vi "SC FPGA.vi"() -> ()   [LabVIEW 2015]
uses:
  <vilib>/eio/EIONode/EIONode.xnode
  <vilib>/rvi/eio/common/nirviEmuTemplateMethod_errors.vi
panel:
  out "Encoder Position":i32
  out "Converted Encoder":bool[](array[boolean])
  out "Raw Encoder":bool[](array[boolean])
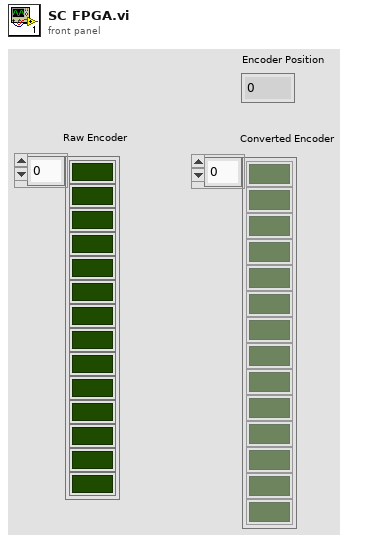
[diagram p1: front panel]
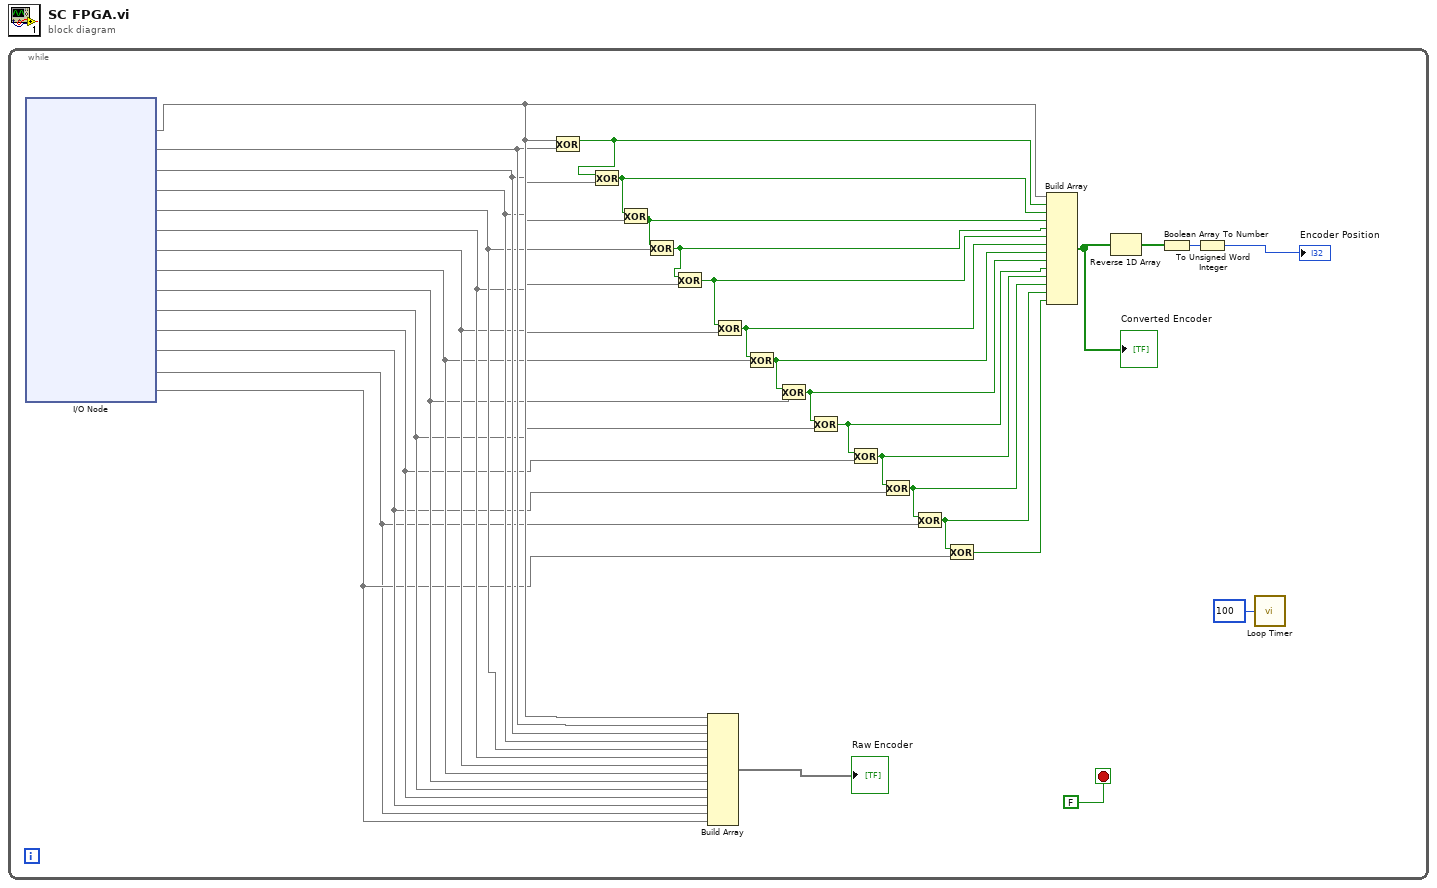
[diagram p0: block diagram]
diagram:
  n1 = while {
    stop <- FALSE stop-if-true
    n2 = xnode "I/O Node"() -> ("Mod6/DIO13"=w15, "Mod6/DIO12"=w14, "Mod6/DIO11"=w13, "Mod6/DIO10"=w12, "Mod6/DIO9"=w11, "Mod6/DIO8"=w10, "Mod6/DIO7"=w9, "Mod6/DIO6"=w8, "Mod6/DIO5"=w7, "Mod6/DIO4"=w6, "Mod6/DIO3"=w5, "Mod6/DIO2"=w4, "Mod6/DIO1"=w2, "Mod6/DIO0"=w3)  [unwired: 14 in, 14 out]
    n3 = Exclusive Or(1:w14, 2:w15) -> (0:w18:bool)
    n4 = Exclusive Or(1:w13, 2:w18) -> (0:w34:bool)
    n5 = Exclusive Or(1:w12, 2:w34) -> (0:w33:bool)
    n6 = Exclusive Or(1:w11, 2:w33) -> (0:w32:bool)
    n7 = Exclusive Or(1:w10, 2:w32) -> (0:w31:bool)
    n8 = Build Array(w15, w14, w13, w12, w11, w10, w9, w8, w7, w6, w5, w4, w2, w3) -> (→"Raw Encoder":void[])
    n9 = Exclusive Or(1:w9, 2:w31) -> (0:w30:bool)
    n10 = Exclusive Or(1:w8, 2:w30) -> (0:w29:bool)
    n11 = Exclusive Or(1:w7, 2:w29) -> (0:w28:bool)
    n12 = Exclusive Or(1:w6, 2:w28) -> (0:w27:bool)
    n13 = Exclusive Or(1:w5, 2:w27) -> (0:w26:bool)
    n14 = Exclusive Or(1:w4, 2:w26) -> (0:w25:bool)
    n15 = Exclusive Or(1:w2, 2:w25) -> (0:w24:bool)
    n16 = Exclusive Or(1:w3, 2:w24) -> (0:w23:bool)
    n17 = Build Array(w15, w18, w34, w33, w32, w31, w30, w29, w28, w27, w26, w25, w24, w23) -> (w21:bool[])
    "Converted Encoder" <- w21
    n18 = Reverse 1D Array(array=w21) -> (reversed array=w22:bool[])
    n19 = Boolean Array To Number(Boolean array=w22) -> (number=w20:u32)
    n20 = To Unsigned Word Integer(number=w20) -> (unsigned 16bit integer=→"Encoder Position":u16)
    n21 = call "Loop Timer"("Count(Ticks)"=u32 100) -> ()  [unwired: 1 out]
  }
